vi "Copy State.vi"(7 "SourceCSM":refnum<class "CSM-Helper.lvclass">=refnum, 8 "error in (no error)":errorcluster, 9 "New(Empty to Use same Name)":string, 10 "Case":string="UI: Cursor Set", 11 "CSM-Helper.lvclass":refnum<class "CSM-Helper.lvclass">=refnum) -> (0 "error out":errorcluster, 3 "CSM-Helper out 2":refnum<class "CSM-Helper.lvclass">)   [LabVIEW 2020, in "CSM-Helper.lvclass"]
uses:
  CSM-Helper.lvclass
  <vilib>/Utility/miscctls.llb/LVPositionTypeDef.ctl
  CSM-Helper.lvclass/CSM-Helper.ctl
  Properties/Read Case Structure Ref.vi
  Get CaseFrame Reference By CaseName.vi
  Properties/Read Block Diagram Ref.vi
  Connect Internal Data Wire If not Connected.vi
  Connect StateQ Wire If not Connected.vi
  Connect Error Wire If not Connected.vi
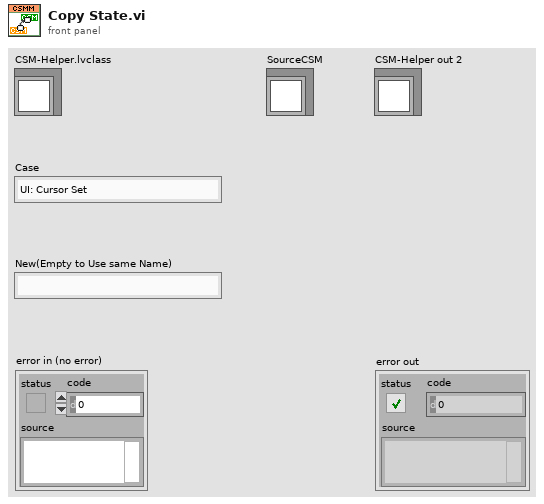
[diagram p1: front panel]
types:
  T1 = typedef "LVPositionTypeDef.ctl" = cluster{"Left":i32, "Top":i32}
  T2 = typedef "LVBoundsTypeDef.ctl" = cluster{"Width":u32, "Height":u32}
  T3 = typedef "CSM-Helper.lvclass/Def-Conncted Information.ctl" = cluster{"Node Index":i32, "Tunnel Relative Pos":T1, "Term Index":i32, "ObjClassName":string, "OwnerClassName":string}
  T4 = cluster{"InternalData":refnum<vi>, "CSM Name":refnum<vi>, "Last Resp":refnum<vi>, "Remaining State":refnum<vi>, "Arguments":refnum<vi>, "Response Source":refnum<vi>, "Source CSM":refnum<vi>, "Selector":refnum<vi>, "Error":refnum<vi>}
  T5 = cluster{"InternalData":refnum<vi>, "Resp":refnum<vi>, "Remaining State":refnum<vi>, "Error":refnum<vi>}
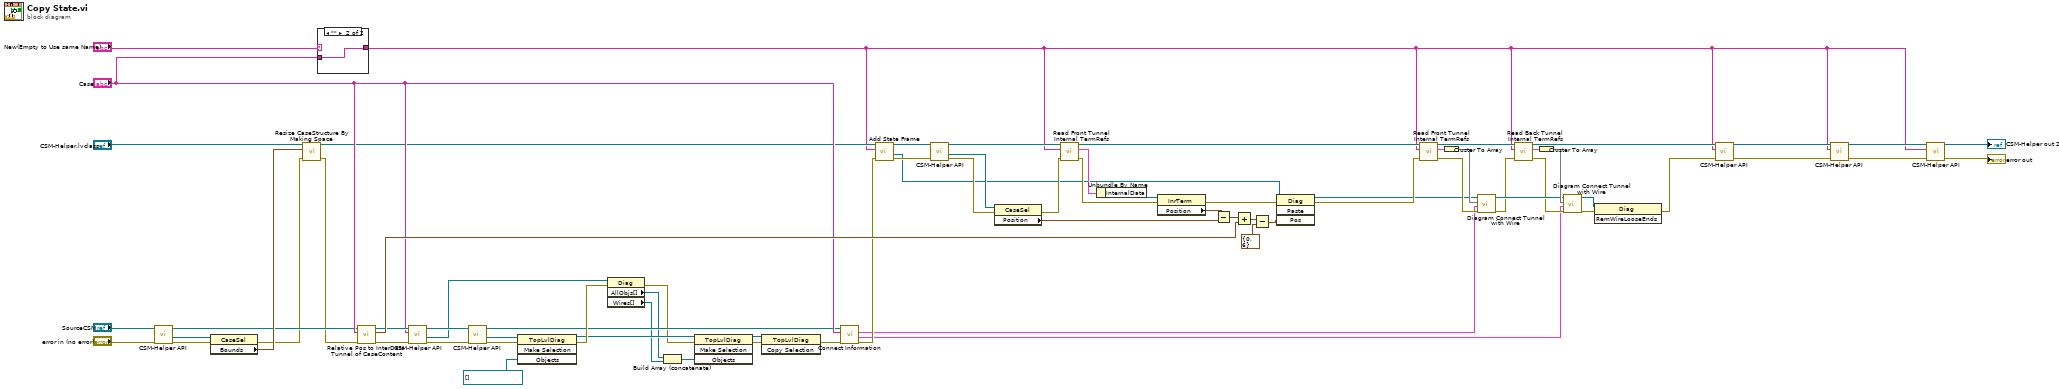
[diagram p0: block diagram]
diagram:
  n1 = call-poly "CSM-Helper API.vi"("error in (no error)"="error in (no error)", "CSM-Helper in"="SourceCSM") -> ("error out"=w25:errorcluster, "Case Structure"=w16:refnum<vi>, "CSM-Helper out"=w22:refnum<class "CSM-Helper.lvclass">)  [unwired: 7 in]
  n2 = property on="Property Node" class="CaseSel"(reference=w16, error in=w25) -> (error out=w21:errorcluster, "Bounds"=w27:T2)  [unwired: 1 out]
  n3 = call "Resize CaseStructure By Making Space.vi"("error in (no error)"=w21, "Bounds"=w27, "CSM-Helper in"="CSM-Helper.lvclass") -> ("error out"=w20:errorcluster, "CSM-Helper out"=w26:refnum<class "CSM-Helper.lvclass">)  [unwired: 5 in, 2 out]
  n4 = case shown="\"\"" "New(Empty to Use same Name)" {
    selector: "New(Empty to Use same Name)" -> [w75 _]
    tunnel: [w75 w76] -> w8
    tunnel: "Case" -> [_ w76]
    frame "False", Default {
    }
    frame "" {
    }
  }
  n5 = call "Relative Pos to InterData Tunnel of CaseContent.vi"("error in (no error)"=w20, "element"="Case", "CSM-Helper in"=w22) -> ("error out"=w36:errorcluster, "Position"=w60:T1, "CSM-Helper out"=w33:refnum<class "CSM-Helper.lvclass">)  [unwired: 6 in]
  n6 = call-poly "CSM-Helper API.vi"("error in (no error)"=w36, "CASE"="Case", "CSM-Helper in"=w33) -> ("error out"=w35:errorcluster, "Frame Refs"=w17:refnum<vi>, "CSM-Helper out"=w34:refnum<class "CSM-Helper.lvclass">)  [unwired: 6 in]
  n7 = call-poly "CSM-Helper API.vi"("error in (no error)"=w35, "CSM-Helper in"=w34) -> ("error out"=w29:errorcluster, "Diagram"=w18:refnum<vi>, "CSM-Helper out"=w13:refnum<class "CSM-Helper.lvclass">)  [unwired: 7 in]
  n8 = invoke on="Invoke Node" class="TopLvlDiag" method="Make Selection"(reference=w18, error in=w29, "Objects"=refnum<vi>[] []) -> (reference out=w7:refnum<vi>, error out=w30:errorcluster)  [unwired: 1 in, 2 out]
  n9 = property class="Diag"(reference=w17, error in=w30) -> (error out=w5:errorcluster, "AllObjs[]"=w3:refnum<vi>[], "Wires[]"=w1:refnum<vi>[])  [unwired: 1 out]
  n10 = Build Array (concatenate)(w3, w1) -> (w2:refnum<vi>[])
  n11 = invoke on="Invoke Node" class="TopLvlDiag" method="Make Selection"(reference=w7, error in=w5, "Objects"=w2) -> (reference out=w6:refnum<vi>, error out=w4:errorcluster)  [unwired: 1 in, 2 out]
  n12 = invoke on="Invoke Node" class="TopLvlDiag" method="Copy Selection"(reference=w6, error in=w4) -> (error out=w38:errorcluster)  [unwired: 1 in, 2 out]
  n13 = call "Connect Information.vi"("error in (no error)"=w38, "Case"="Case", "CSM-Helper in"=w13) -> ("error out"=w37:errorcluster, "Backend Connected Info"=w11:T3[], "FrontEnd Connected Info"=w12:T3[])  [unwired: 5 in, 1 out]
  n14 = call "Add State Frame.vi"("error in (no error)"=w37, "element"=w8, "CSM-Helper in"=w26) -> ("error out"=w67:errorcluster, "Add Frame"=w14:refnum<vi>, "CSM-Helper out"=w73:refnum<class "CSM-Helper.lvclass">)  [unwired: 6 in]
  n15 = call-poly "CSM-Helper API.vi"("error in (no error)"=w67, "CSM-Helper in"=w73) -> ("error out"=w40:errorcluster, "Case Structure"=w15:refnum<vi>, "CSM-Helper out"=w68:refnum<class "CSM-Helper.lvclass">)  [unwired: 7 in]
  n16 = property on="Property Node" class="CaseSel"(reference=w15, error in=w40) -> (error out=w39:errorcluster, "Position"=w63:T1)  [unwired: 1 out]
  n17 = call "Read Front Tunnel Internal TermRefs.vi"("error in (no error)"=w39, "case"=w8, "CSM-Helper in"=w68) -> ("error out"=w71:errorcluster, "Front Tunnels"=w70:T4, "CSM-Helper out"=w69:refnum<class "CSM-Helper.lvclass">)  [unwired: 6 in]
  n18 = Unbundle By Name(w70) -> ("InternalData"=w74:refnum<vi>)
  n19 = property on="Property Node" class="InrTerm"(reference=w74, error in=w71) -> (error out=w72:errorcluster, "Position"=w64:T1)  [unwired: 1 out]
  n20 = Subtract(x=w64, y=w63) -> (x-y=w66:T1)
  n21 = Add(x=w66, y=w60) -> (x+y=w65:T1)
  n22 = Subtract(x=w65, y=T1 {"Left"=0, "Top"=6}) -> (x-y=w62:T1)
  n23 = invoke on="Invoke Node" class="Diag" method="Paste"(reference=w14, error in=w72, "Pos"=w62) -> (reference out=w9:refnum<vi>, error out=w10:errorcluster)  [unwired: 1 in, 2 out]
  n24 = call "Read Front Tunnel Internal TermRefs.vi"("error in (no error)"=w10, "case"=w8, "CSM-Helper in"=w69) -> ("error out"=w58:errorcluster, "Front Tunnels"=w57:T4, "CSM-Helper out"=w55:refnum<class "CSM-Helper.lvclass">)  [unwired: 6 in]
  n25 = Cluster To Array(cluster=w57) -> (array=w59:refnum<vi>[])
  n26 = call "Diagram Connect Tunnel with Wire.vi"("error in (no error)"=w58, "FrontEnd Connected Info"=w12, "Front Tunnels"=w59, "Diagram in"=w9) -> ("error out"=w48:errorcluster, "Diagram out"=w50:refnum<vi>)  [unwired: 5 in, 1 out]
  n27 = call "Read Back Tunnel Internal TermRefs.vi"("error in (no error)"=w48, "element"=w8, "CSM-Helper in"=w55) -> ("error out"=w47:errorcluster, "Front Tunnels"=w56:T5, "CSM-Helper out"=w54:refnum<class "CSM-Helper.lvclass">)  [unwired: 6 in]
  n28 = Cluster To Array(cluster=w56) -> (array=w51:refnum<vi>[])
  n29 = call "Diagram Connect Tunnel with Wire.vi"("error in (no error)"=w47, "FrontEnd Connected Info"=w11, "Front Tunnels"=w51, "Diagram in"=w50) -> ("error out"=w49:errorcluster, "Diagram out"=w43:refnum<vi>)  [unwired: 5 in, 1 out]
  n30 = invoke on="Invoke Node" class="Diag" method="RemWireLooseEnds"(reference=w43, error in=w49) -> (error out=w44:errorcluster)  [unwired: 1 in, 2 out]
  n31 = call-poly "CSM-Helper API.vi"("error in (no error)"=w44, "case"=w8, "CSM-Helper in"=w54) -> ("error out"=w53:errorcluster, "CSM-Helper out"=w52:refnum<class "CSM-Helper.lvclass">)  [unwired: 7 in]
  n32 = call-poly "CSM-Helper API.vi"("error in (no error)"=w53, "case"=w8, "CSM-Helper in"=w52) -> ("error out"=w45:errorcluster, "CSM-Helper out"=w46:refnum<class "CSM-Helper.lvclass">)  [unwired: 7 in]
  n33 = call-poly "CSM-Helper API.vi"("error in (no error)"=w45, "case"=w8, "CSM-Helper in"=w46) -> ("error out"=→"error out":errorcluster, "CSM-Helper out"=→"CSM-Helper out 2":refnum<class "CSM-Helper.lvclass">)  [unwired: 7 in]
